vi "DMA-Ch-5761.vi"(4 "DMATtoHOST":refnum<k21>="DMATtoHOST0", 5 "IntermediateFIFO":refnum<k21>="FIFO0", 6 "ProcessingFIFO":refnum<k21>="Processing0", 7 "AI Cluster":T1={"FPGA AI3"="IO Module\\AI 0 Data N", "FPGA AI3 2"="IO Module\\AI 1 Data N", "FPGA AI3 3"="IO Module\\AI 2 Data N", "FPGA AI3 4"="IO Module\\AI 3 Data N"}, 8 "Processing":bool, 9 "Nchannels":T2=enum."4 Channels", 10 "Source Name":refnum<k21>="100 MHz Clock", 11 "DMA number":i16) -> ()   [LabVIEW 2013]
uses:
  N Channels 5761.ctl
  StateControl.ctl
  <vilib>/Platform/TimedLoop/XDataNode/timing_clust.ctl
  <vilib>/Platform/TimedLoop/XDataNode/nitl_modes.ctl
  <vilib>/Platform/TimedLoop/XDataNode/wakeup.ctl
  <vilib>/rvi/Emulation/niFpgaSctlEmulationGetInTimedLoop.vi
  <vilib>/rvi/Emulation/niFpgaEmulationReportErrorSimple.vi
  <vilib>/rvi/Emulation/niFpgaGetClockAttributes.vi
  <vilib>/rvi/Emulation/niFpgaCriticalErrorInLSC.vi
  <vilib>/rvi/DataTransferAndStorage/Container/Common/niFpgaContainerExecOnDevCompGetState.vi
  <vilib>/rvi/FIFO/Fifo_Resource/nirvififoEmulationGetNumberOfElementsToReadFpgaImpl.vi
  <vilib>/rvi/DataTransferAndStorage/Container/Common/niFpgaContainerGetUniqueNameForEmu.vi
  <vilib>/rvi/interface/RandomDataEmulation/nirviRandomDataFPGAFIFO.vi
  <vilib>/rvi/interface/RandomDataEmulation/niFpgaRandomDataHandleErrors.vi
  <vilib>/rvi/eio/common/nirviEmuReportErrorAndStop.vi
  <vilib>/rvi/FIFO/Fifo_Resource/nirvififoEmulationReadFpgaImpl.vi
  <vilib>/rvi/FIFO/Fifo_Resource/nirvififoEmulationWriteFpgaImpl.vi
  <vilib>/rvi/Emulation/niFpgaProcessEmulError.vi
  GlobalReg.vi
  <vilib>/Platform/TimedLoop/XDataNode/XDataNode.xnode
  <vilib>/rvi/DataTransferAndStorage/Container/XNode/niFpgaContainer.xnode
  <vilib>/rvi/FIFO/Fifo_Resource/niFpgaFifoEmulationRefIn.vi
  <vilib>/rvi/interface/RandomDataEmulation/nirviRandomDataFpgaReadWriteTemplate.vi
  <vilib>/Platform/TimedLoop/XDataNode/XDNodeRunTimeDep.lvlib
panel:
  in  "DebugMode":bool
  in  "DAQStartStop":bool
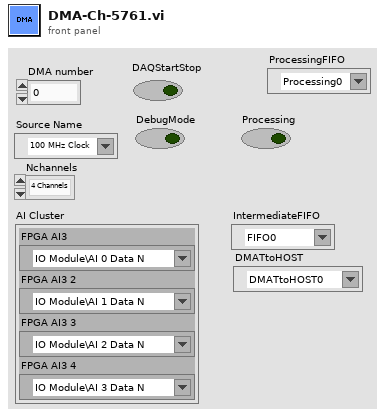
[diagram p1: front panel]
types:
  T1 = cluster{"FPGA AI3":refnum<k21>, "FPGA AI3 2":refnum<k21>, "FPGA AI3 3":refnum<k21>, "FPGA AI3 4":refnum<k21>}
  T2 = typedef "N Channels 5761.ctl" = enum16{"0 Channels", "1 Channels", "2 Channels", "3 Channels", "4 Channels", ""}
  T3 = typedef "StateControl.ctl" = enum16{"Idle", "Acq"}
  T4 = typedef "XDNodeRunTimeDep.lvlib/timing_clust.ctl" = cluster{"Expected End [f-1]":u64, "Actual End [f-1]":u64, "Finished Late? [f-1]":bool, "Expected End [i-1]":u64, "Actual End [i-1]":u64, "Finished Late? [i-1]":bool, "Expected Start [i]":u64, "Actual Start [i]":u64, "Expected Start [f]":u64, "Actual Start [f]":u64, "Source Name":string, "Structure Name":string, "Period":i64, "Deadline":i64, "Offset":i64, "Start":i64, "Priority":i32, "Timeout":i32, "Mode":T5, "Wakeup Reason":T6, "Error":errorcluster, "Source Type":string, "Secondary Source Type":string, "Global End Time":u64, "Global Start Time":u64, "Frame Duration":u64, "Iteration Duration":u64, "Assigned CPU":i32, "I/O Scan Engine Mode":u32}
  T5 = typedef "XDNodeRunTimeDep.lvlib/nitl_modes.ctl" = enum32{"No Change", "Process missed periods, maintain original phase", "Discard missed periods, maintain original phase", "Process missed periods, ignore original phase", "Discard missed periods, ignore original phase"}
  T6 = typedef "XDNodeRunTimeDep.lvlib/wakeup.ctl" = enum32{"Normal", "Aborted", "Asynchronous wakeup", "Timing source error", "Timed loop error", "Timeout"}
  T7 = cluster{u16, u16, u64, u64, u64, u64, i16, bool, bool, u64, u16, u16}
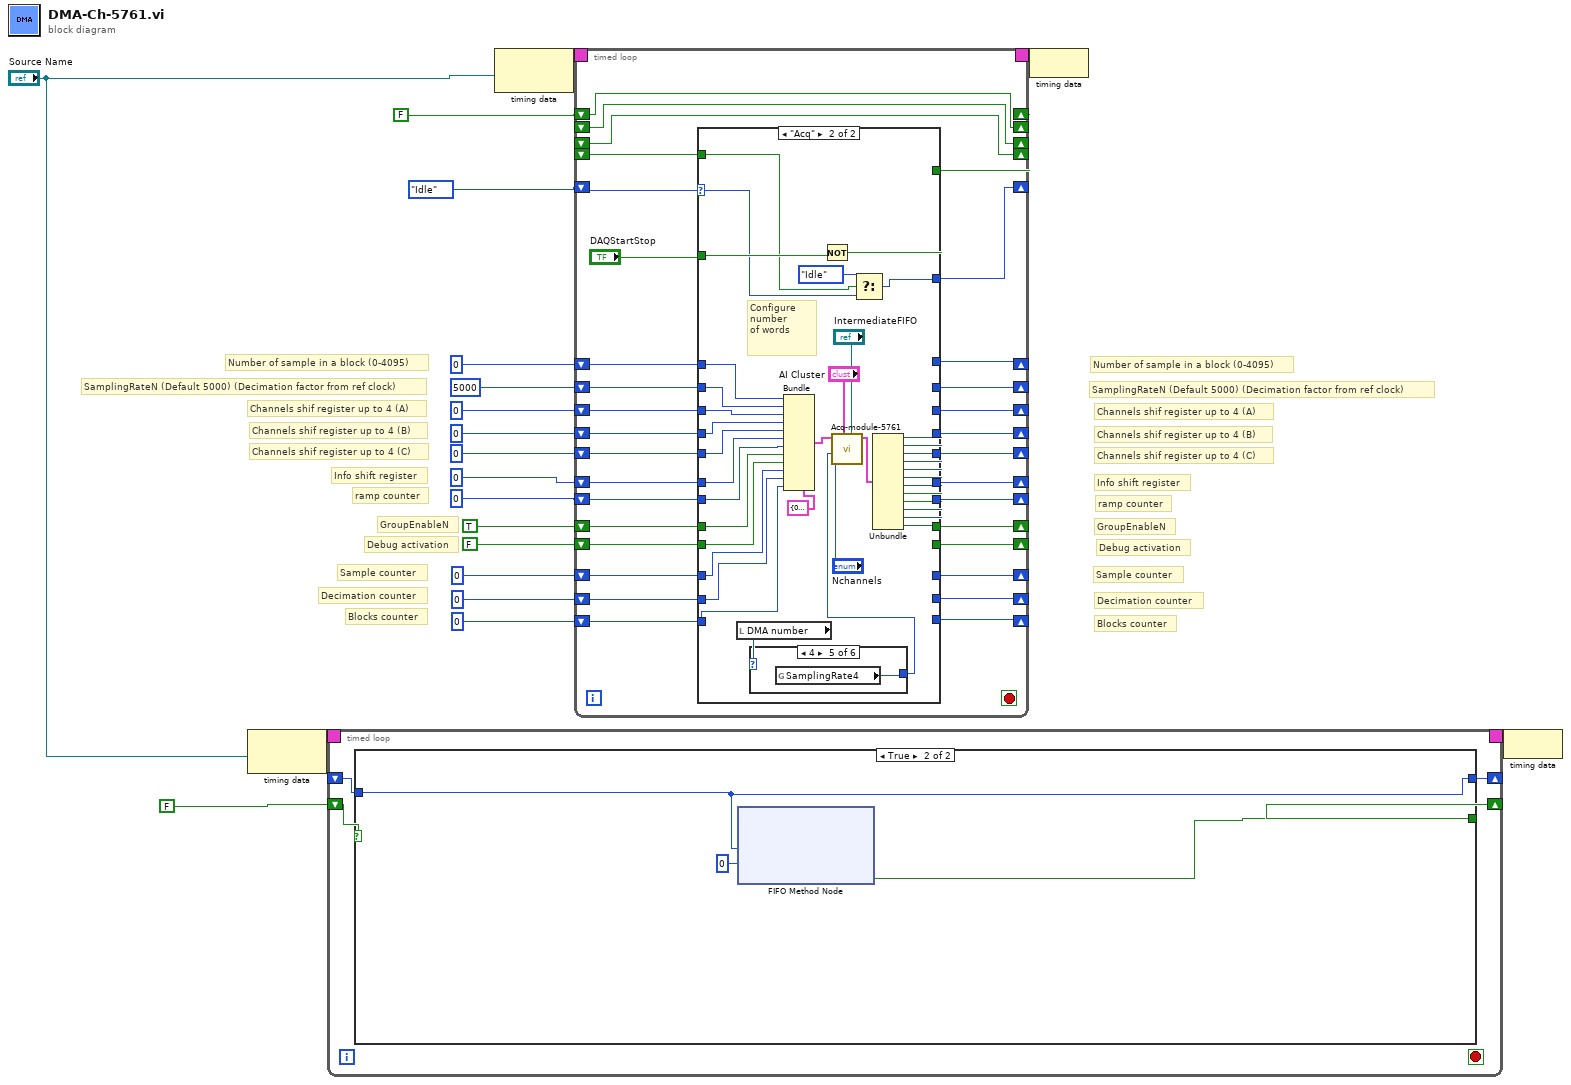
[diagram p0: block diagram]
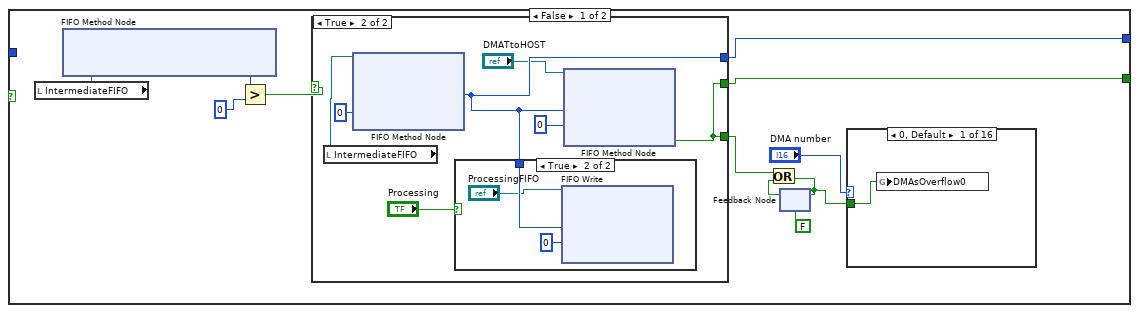
[diagram p2: hidden frame]
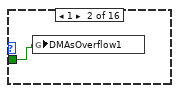
[diagram p3: hidden frame]
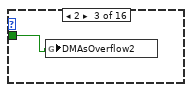
[diagram p4: hidden frame]
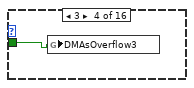
[diagram p5: hidden frame]
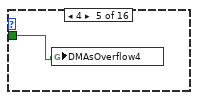
[diagram p6: hidden frame]
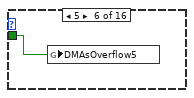
[diagram p7: hidden frame]
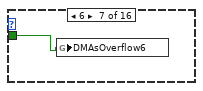
[diagram p8: hidden frame]
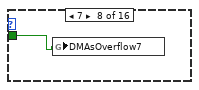
[diagram p9: hidden frame]
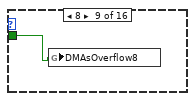
[diagram p10: hidden frame]
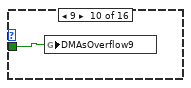
[diagram p11: hidden frame]
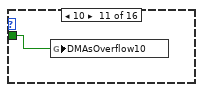
[diagram p12: hidden frame]
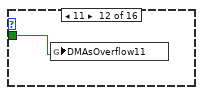
[diagram p13: hidden frame]
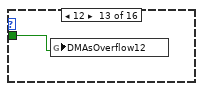
[diagram p14: hidden frame]
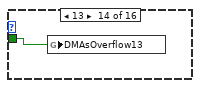
[diagram p15: hidden frame]
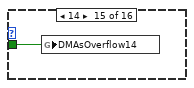
[diagram p16: hidden frame]
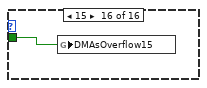
[diagram p17: hidden frame]
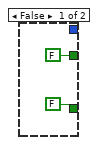
[diagram p18: hidden frame]
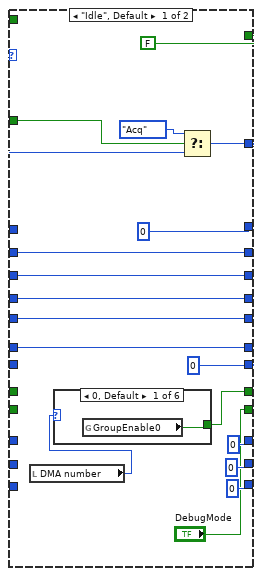
[diagram p20: hidden frame]
diagram:
  # "Blocks counter"
  # "Decimation counter"
  # "Sample counter"
  # "Debug activation"
  # "ramp counter"
  # "Info shift register"
  # "Channels shif register up to 4 (C)"
  # "Channels shif register up to 4 (B)"
  # "Channels shif register up to 4 (A)"
  # "SamplingRateN (Default 5000) (Decimation factor from ref clock)"
  # "Number of sample in a block (0-4095)"
  # "GroupEnableN"
  # "Blocks counter"
  # "Decimation counter"
  # "Sample counter"
  # "Debug activation"
  # "ramp counter"
  # "Info shift register"
  # "Channels shif register up to 4 (C)"
  # "Channels shif register up to 4 (B)"
  # "Channels shif register up to 4 (A)"
  # "SamplingRateN (Default 5000) (Decimation factor from ref clock)"
  # "Number of sample in a block (0-4095)"
  # "GroupEnableN"
  n1 = node-c288("Source Name") -> (w4:T4)
  n2 = timed-loop {
    timing: w4 -> [_]
    timing-out: [_] -> w3
    shift-right: [w24] -> _
    shift-left: FALSE ("Timed Out?") -> [w23]
    shift-right: [w21] -> _
    shift-left: _ -> [w22]
    stop <- _ stop-if-true
    n3 = case shown="True" w23 {
      tunnel: [w28 w65] -> w24
      tunnel: w22 -> [_ w64]
      tunnel: [w29 w64] -> w21
      frame False {
        n4 = local read "IntermediateFIFO"() -> (w25:refnum<k21>)
        n5 = xnode ("FIFO Method Node")("FIFO In"=w25) -> ("Number of Elements to Read"=w35:u32)  [unwired: 1 out]
        n6 = Greater?(x=w35, y=u32 0) -> (0:w33:bool)
        n7 = case shown="True" w33 {
          tunnel: [FALSE ("Timed Out?") w58] -> w30
          tunnel: [FALSE ("Timed Out?") w58] -> w28
          tunnel: [_ w57] -> w29
          frame False {
          }
          frame True {
            n8 = local read "IntermediateFIFO"() -> (w55:refnum<k21>)
            n9 = xnode ("FIFO Method Node")("Timeout"=0, "FIFO In"=w55) -> ("Element"=w57:u64)  [unwired: 2 out]
            n10 = case shown="True" "Processing" {
              tunnel: w57 -> [_ w62]
              frame False {
              }
              frame True {
                n11 = xnode "FIFO Write"("Element"=w62, "Timeout"=0, "FIFO In"="ProcessingFIFO") -> ()  [unwired: 2 out]
              }
            }
            n12 = xnode ("FIFO Method Node")("Element"=w57, "Timeout"=0, "FIFO In"="DMATtoHOST") -> ("Timed Out?"=w58:bool)  [unwired: 1 out]
          }
        }
        n13 = feedback #1(FALSE) -> (w31:bool)
        n14 = Or(x=w30, y=w31) -> (x .or. y?=w27:bool)
        n15 = feedback-in #1(w27) -> ()
        n16 = case shown="0, Default" "DMA number" {
          tunnel: w27 -> [w36 w37 w38 w39 w40 w41 w42 w43 w44 w45 w46 w47 w48 w49 w50 w51]
          frame 0, Default {
            n17 = global write "GlobalReg.vi" "DMAsOverflow0"(w36) -> ()
          }
          frame 1 {
            n18 = global write "GlobalReg.vi" "DMAsOverflow1"(w37) -> ()
          }
          frame 2 {
            n19 = global write "GlobalReg.vi" "DMAsOverflow2"(w38) -> ()
          }
          frame 3 {
            n20 = global write "GlobalReg.vi" "DMAsOverflow3"(w39) -> ()
          }
          frame 4 {
            n21 = global write "GlobalReg.vi" "DMAsOverflow4"(w40) -> ()
          }
          frame 5 {
            n22 = global write "GlobalReg.vi" "DMAsOverflow5"(w41) -> ()
          }
          frame 6 {
            n23 = global write "GlobalReg.vi" "DMAsOverflow6"(w42) -> ()
          }
          frame 7 {
            n24 = global write "GlobalReg.vi" "DMAsOverflow7"(w43) -> ()
          }
          frame 8 {
            n25 = global write "GlobalReg.vi" "DMAsOverflow8"(w44) -> ()
          }
          frame 9 {
            n26 = global write "GlobalReg.vi" "DMAsOverflow9"(w45) -> ()
          }
          frame 10 {
            n27 = global write "GlobalReg.vi" "DMAsOverflow10"(w46) -> ()
          }
          frame 11 {
            n28 = global write "GlobalReg.vi" "DMAsOverflow11"(w47) -> ()
          }
          frame 12 {
            n29 = global write "GlobalReg.vi" "DMAsOverflow12"(w48) -> ()
          }
          frame 13 {
            n30 = global write "GlobalReg.vi" "DMAsOverflow13"(w49) -> ()
          }
          frame 14 {
            n31 = global write "GlobalReg.vi" "DMAsOverflow14"(w50) -> ()
          }
          frame 15 {
            n32 = global write "GlobalReg.vi" "DMAsOverflow15"(w51) -> ()
          }
        }
      }
      frame True {
        n33 = xnode ("FIFO Method Node")("Element"=w64, "Timeout"=0) -> ("Timed Out?"=w65:bool)  [unwired: 1 in, 1 out]
      }
    }
  }
  n34 = node-c288("Source Name") -> (w20:T4)
  n35 = timed-loop {
    timing: w20 -> [_]
    timing-out: [_] -> w19
    shift-right: [w98] -> _
    shift-left: StateControl."Idle" ("Enum") -> [w100]
    shift-right: [w96] -> _
    shift-left: u16 0 ("sample of block out") -> [w97]
    shift-right: [w94] -> _
    shift-left: u16 5000 ("FS1") -> [w95]
    shift-right: [w92] -> _
    shift-left: u64 0 -> [w93]
    shift-right: [w90] -> _
    shift-left: u64 0 -> [w91]
    shift-right: [w88] -> _
    shift-left: u64 0 -> [w89]
    shift-right: [w86] -> _
    shift-left: u64 0 ("Element") -> [w87]
    shift-right: [w69] -> _
    shift-left: i16 0 -> [w85]
    shift-right: [w75] -> _
    shift-left: TRUE ("DMA1activation") -> [w84]
    shift-right: [w76] -> _
    shift-left: FALSE -> [w83]
    shift-right: [w79] -> _
    shift-left: u64 0 ("contador muestra") -> [w82]
    shift-right: [w78] -> _
    shift-left: u16 0 -> [w81]
    shift-right: [w77] -> _
    shift-left: u16 0 -> [w80]
    shift-right: [w74] -> _
    shift-left: FALSE -> [w73]
    shift-right: [w73] -> _
    shift-left: _ -> [w72]
    shift-right: [w72] -> _
    shift-left: _ -> [w71]
    shift-right: [w71] -> _
    shift-left: _ -> [w70]
    stop <- _ stop-if-true
    n36 = case shown="\"Acq\"" w100 {
      selector: w100 -> [w116 w158]
      tunnel: "DAQStartStop" -> [w118 w162]
      tunnel: [w115 w157] -> w98
      tunnel: w97 -> [_ w155]
      tunnel: [u16 0 ("sample of block out") w143] -> w96
      tunnel: w95 -> [w113 w154]
      tunnel: [w113 w142] -> w94
      tunnel: w93 -> [w112 w153]
      tunnel: [w112 w141] -> w92
      tunnel: w91 -> [w111 w152]
      tunnel: [w111 w140] -> w90
      tunnel: w89 -> [w110 w151]
      tunnel: [w110 w139] -> w88
      tunnel: w87 -> [w109 w150]
      tunnel: [w109 w138] -> w86
      tunnel: w85 -> [_ w149]
      tunnel: w84 -> [_ w148]
      tunnel: w83 -> [_ w147]
      tunnel: w82 -> [_ w146]
      tunnel: w81 -> [_ w145]
      tunnel: w80 -> [_ w144]
      tunnel: [u64 0 ("contador muestra") w134] -> w79
      tunnel: [u16 0 w133] -> w78
      tunnel: [u16 0 w132] -> w77
      tunnel: ["DebugMode" w135] -> w76
      tunnel: [w102 w136] -> w75
      tunnel: [FALSE w161] -> w74
      tunnel: w70 -> [_ w160]
      tunnel: [i16 0 w137] -> w69
      frame "Idle", Default {
        n37 = local read "DMA number"() -> (w101:i16)
        n38 = case shown="0, Default" w101 {
          tunnel: [w119 w120 w121 w122 w123 w124] -> w102
          frame 0, Default {
            n39 = global read "GlobalReg.vi" "GroupEnable0"() -> (w119:bool)
          }
          frame 1 {
            n40 = global read "GlobalReg.vi" "GroupEnable1"() -> (w120:bool)
          }
          frame 2 {
            n41 = global read "GlobalReg.vi" "GroupEnable2"() -> (w121:bool)
          }
          frame 3 {
            n42 = global read "GlobalReg.vi" "GroupEnable3"() -> (w122:bool)
          }
          frame 4 {
            n43 = global read "GlobalReg.vi" "GroupEnable4"() -> (w123:bool)
          }
          frame 5 {
            n44 = global read "GlobalReg.vi" "GroupEnable5"() -> (w124:bool)
          }
        }
        n45 = Select(t=StateControl."Acq" ("Enum"), s=w118, f=w116) -> (s? t:f=w115:T3)
      }
      frame "Acq" {
        # "Configure number \nof words"
        n46 = local read "DMA number"() -> (w127:i16)
        n47 = case shown="4" w127 {
          tunnel: [w163 w164 w165 w166 w167 w168] -> w126
          frame 0, Default {
            n48 = global read "GlobalReg.vi" "SamplingRate0"() -> (w163:u16)
          }
          frame 1 {
            n49 = global read "GlobalReg.vi" "SamplingRate1"() -> (w164:u16)
          }
          frame 2 {
            n50 = global read "GlobalReg.vi" "SamplingRate2"() -> (w165:u16)
          }
          frame 3 {
            n51 = global read "GlobalReg.vi" "SamplingRate3"() -> (w166:u16)
          }
          frame 4 {
            n52 = global read "GlobalReg.vi" "SamplingRate4"() -> (w167:u16)
          }
          frame 5 {
            n53 = global read "GlobalReg.vi" "SamplingRate5"() -> (w168:u16)
          }
        }
        n54 = Bundle(cluster=T7 {0, 0, 0, 0, 0, 0, 0, TRUE, TRUE, 0, 0, 0} ("Cluster in"), w155, w154, w153, w152, w151, w150, w149, w148, w147, w146, w145, w144) -> (w131:T7)
        n55 = Not(x=w162) -> (.not. x?=w161:bool)
        n56 = call "Acq-module-5761.vi"("IntermediateFIFO"="IntermediateFIFO", "AI Cluster"="AI Cluster", "Nchannels"="Nchannels", "SamplingRate0"=w126, "Cluster in"=w131) -> ("cluster out"=w130:T7)  [unwired: 5 in, 1 out]
        n57 = Select(t=StateControl."Idle" ("Enum"), s=w160, f=w158) -> (s? t:f=w157:T3)
        n58 = Unbundle(w130) -> (w143:u16, w142:u16, w141:u64, w140:u64, w139:u64, w138:u64, w137:i16, w136:bool, w135:bool, w134:u64, w133:u16, w132:u16)
      }
    }
  }
  n59 = node-c288(w19) -> ()
  n60 = node-c288(w3) -> ()
